vi "WaitforWLM_example_2017.vi"() -> ()   [LabVIEW 2017]
uses:
  wlmData.dll
panel:
  out "error out":errorcluster
  out "Power":dbl
  out "power graph":dbl[](graph)
  out "wavelength graph":dbl[](graph)
  in  "stop":bool
  out "wavelength / nm":dbl format="%#_18f"
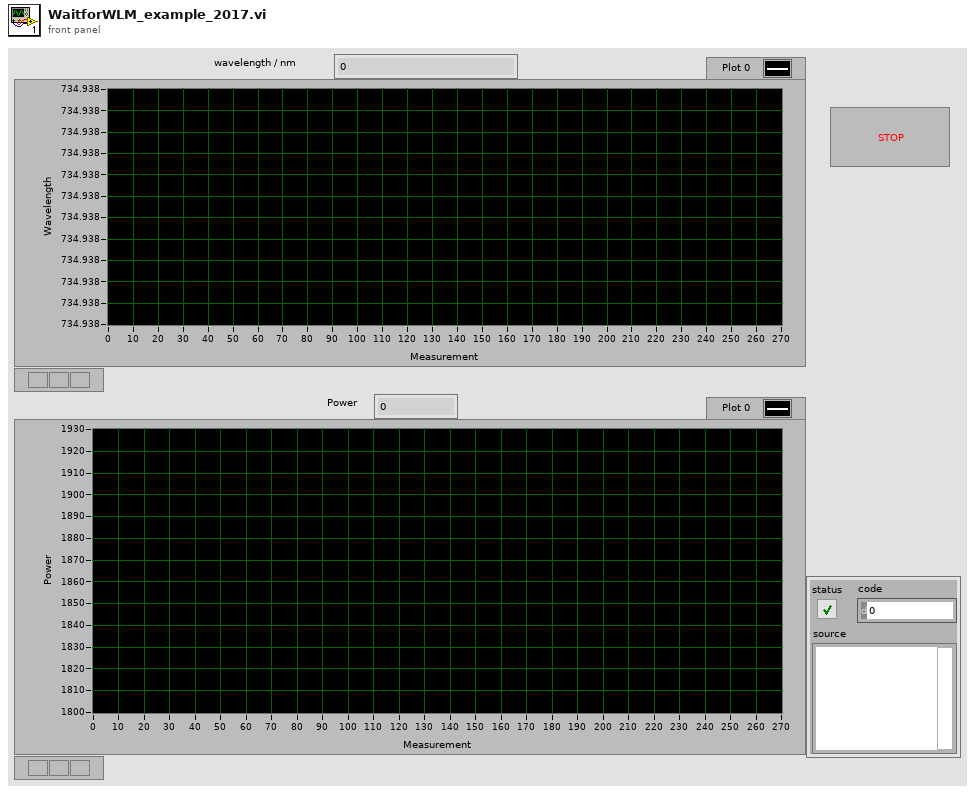
[diagram p1: front panel]
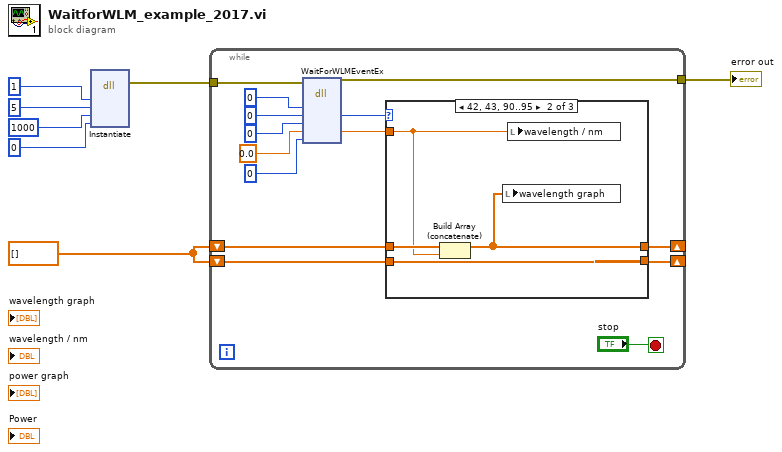
[diagram p0: block diagram]
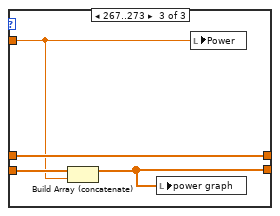
[diagram p3: hidden frame]
diagram:
  w1 = dbl[] []
  n1 = dll-call lib="wlmData.dll" fn="Instantiate"("arg1"=u32 1, "arg2"=5, "arg3"=u32 1000, "arg4"=u32 0) -> (error out=w4:errorcluster)  [unwired: 8 in, 1 out]
  n2 = while {
    tunnel: w4 -> [w15]
    shift-right: [w12] -> _
    shift-left: w1 -> [w11]
    tunnel: [w10] -> w2
    shift-right: [w8] -> _
    shift-left: w1 -> [w9]
    stop <- "stop" stop-if-true
    n3 = dll-call lib="wlmData.dll" fn="WaitForWLMEventEx"(error in=w15, "Ver"=0, "Mode"=0, "IntVal"=0, "DblVal"=0.0, "Res"=0) -> (error out=w10:errorcluster, "Mode"=w14:i32, "DblVal"=w13:dbl)  [unwired: 6 in, 1 out]
    n4 = case shown="42, 43, 90..95" w14 {
      tunnel: w13 -> [_ w25 w28]
      tunnel: w11 -> [w23 w27 w30]
      tunnel: [w23 w26 w30] -> w12
      tunnel: w9 -> [w22 w24 w31]
      tunnel: [w22 w24 w29] -> w8
      frame 0, Default {
      }
      frame 42, 43, 90..95 {
        n5 = Build Array (concatenate)(w27, w25) -> (w26:dbl[])
        n6 = local write "wavelength graph"(w26) -> ()
        n7 = local write "wavelength / nm"(w25) -> ()
      }
      frame 267..273 {
        n8 = Build Array (concatenate)(w31, w28) -> (w29:dbl[])
        n9 = local write "power graph"(w29) -> ()
        n10 = local write "Power"(w28) -> ()
      }
    }
  }
  "error out" <- w2
